vi "SP_BreakDown_Manage.vi"() -> ()   [LabVIEW 2017]
uses:
  <vilib>/addons/database/Connection.llb/DB Tools Open Connec (Path).vi
  Globle/Login Data.vi
  <vilib>/addons/database/NI_Database_API.lvlib
panel:
  in  "Cancel Button - Archive":bool
  out "Stakeholder":string
  out "Role Id":string
  in  "Download 2":bool
  in  "Get Rport 2":bool
  in  "Manage 2":bool
  out "Table 2":string[][](array[string])
  out "error out":errorcluster
  in  "error in (no error)":errorcluster
  out "Table":string[][](table)
  in  "Shift":string(combo)
  in  "Station":string(combo)
  in  "To Date":timestamp format="%<%Y-%m-%d>T"
  in  "From Date":timestamp format="%<%Y-%m-%d>T"
  in  "Stakeholder":string(combo)
  # "Breakdown Manage"
  # "Designed And Developed By - Infinity Automation Systems Pvt. Ltd."
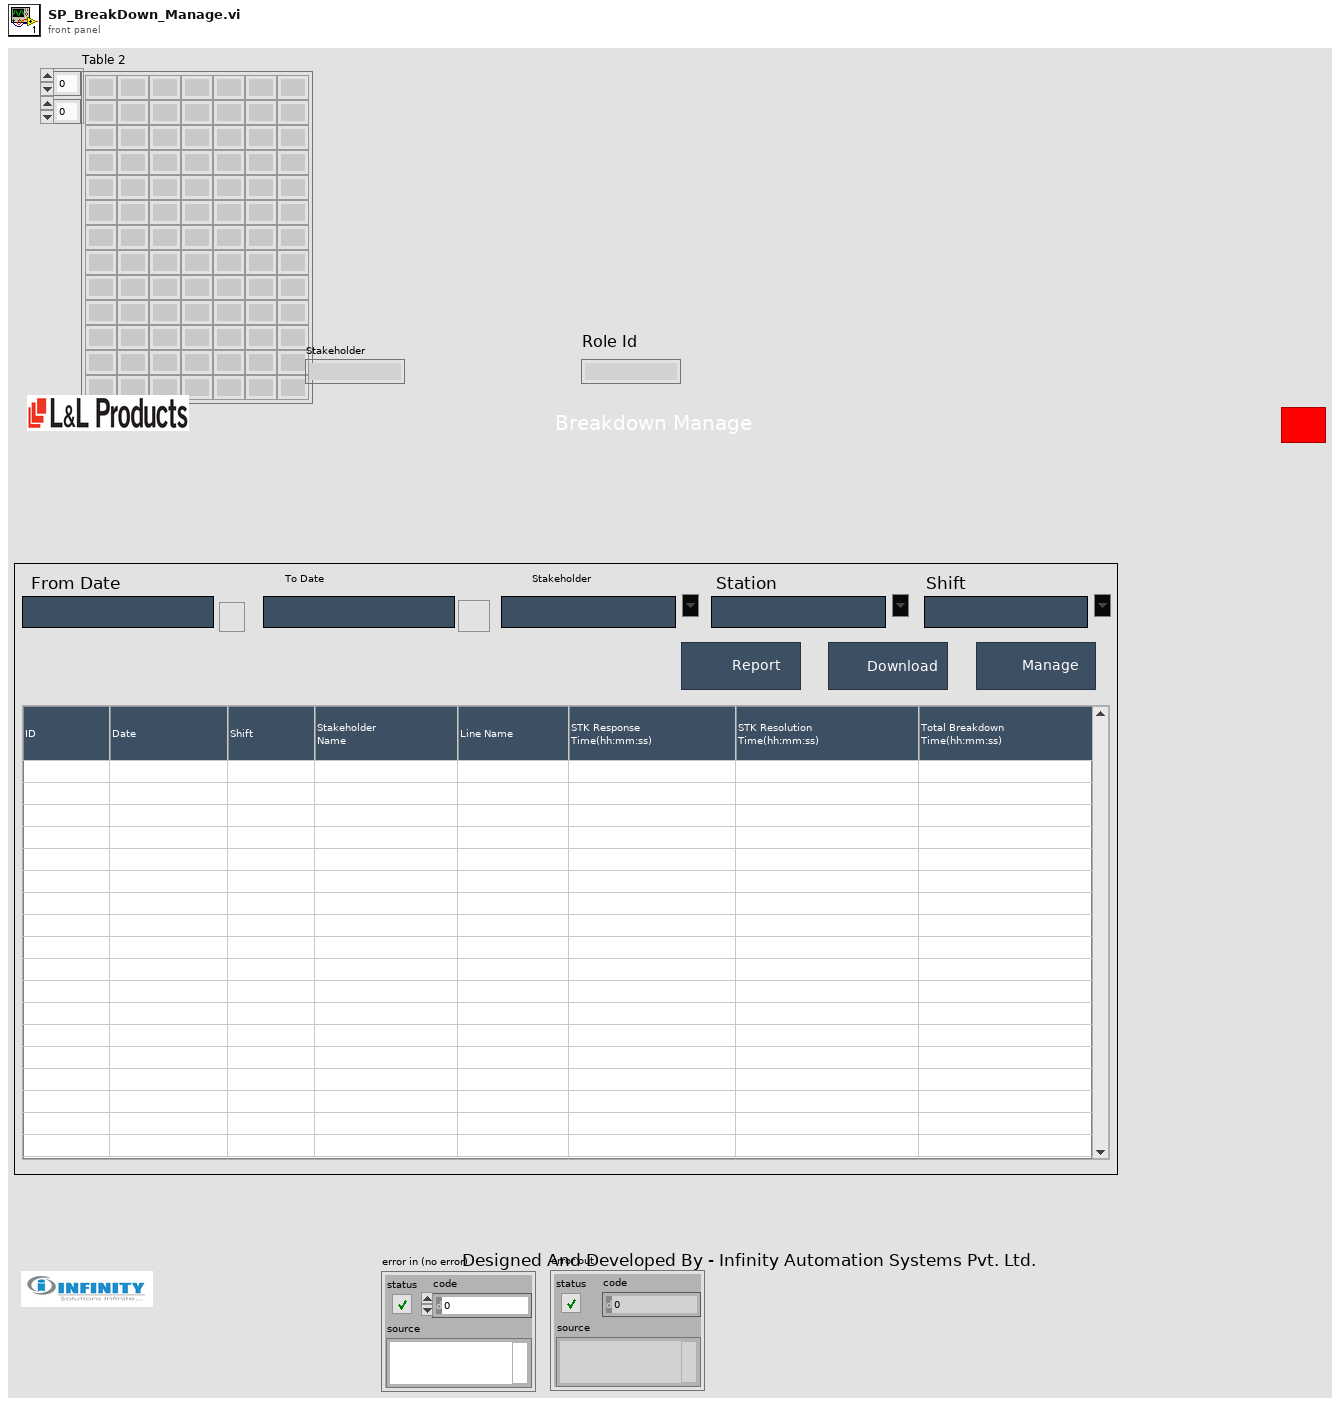
[diagram p1: front panel]
types:
  T1 = typedef "NI_Database_API.lvlib/Conn ObjectReference.ctl" = refnum<k1>
  T2 = enum32{"invalid app kind", "Development System", "Run Time System", "Student Edition", "Embedded LabVIEW", "Evaluation", "Custom"}
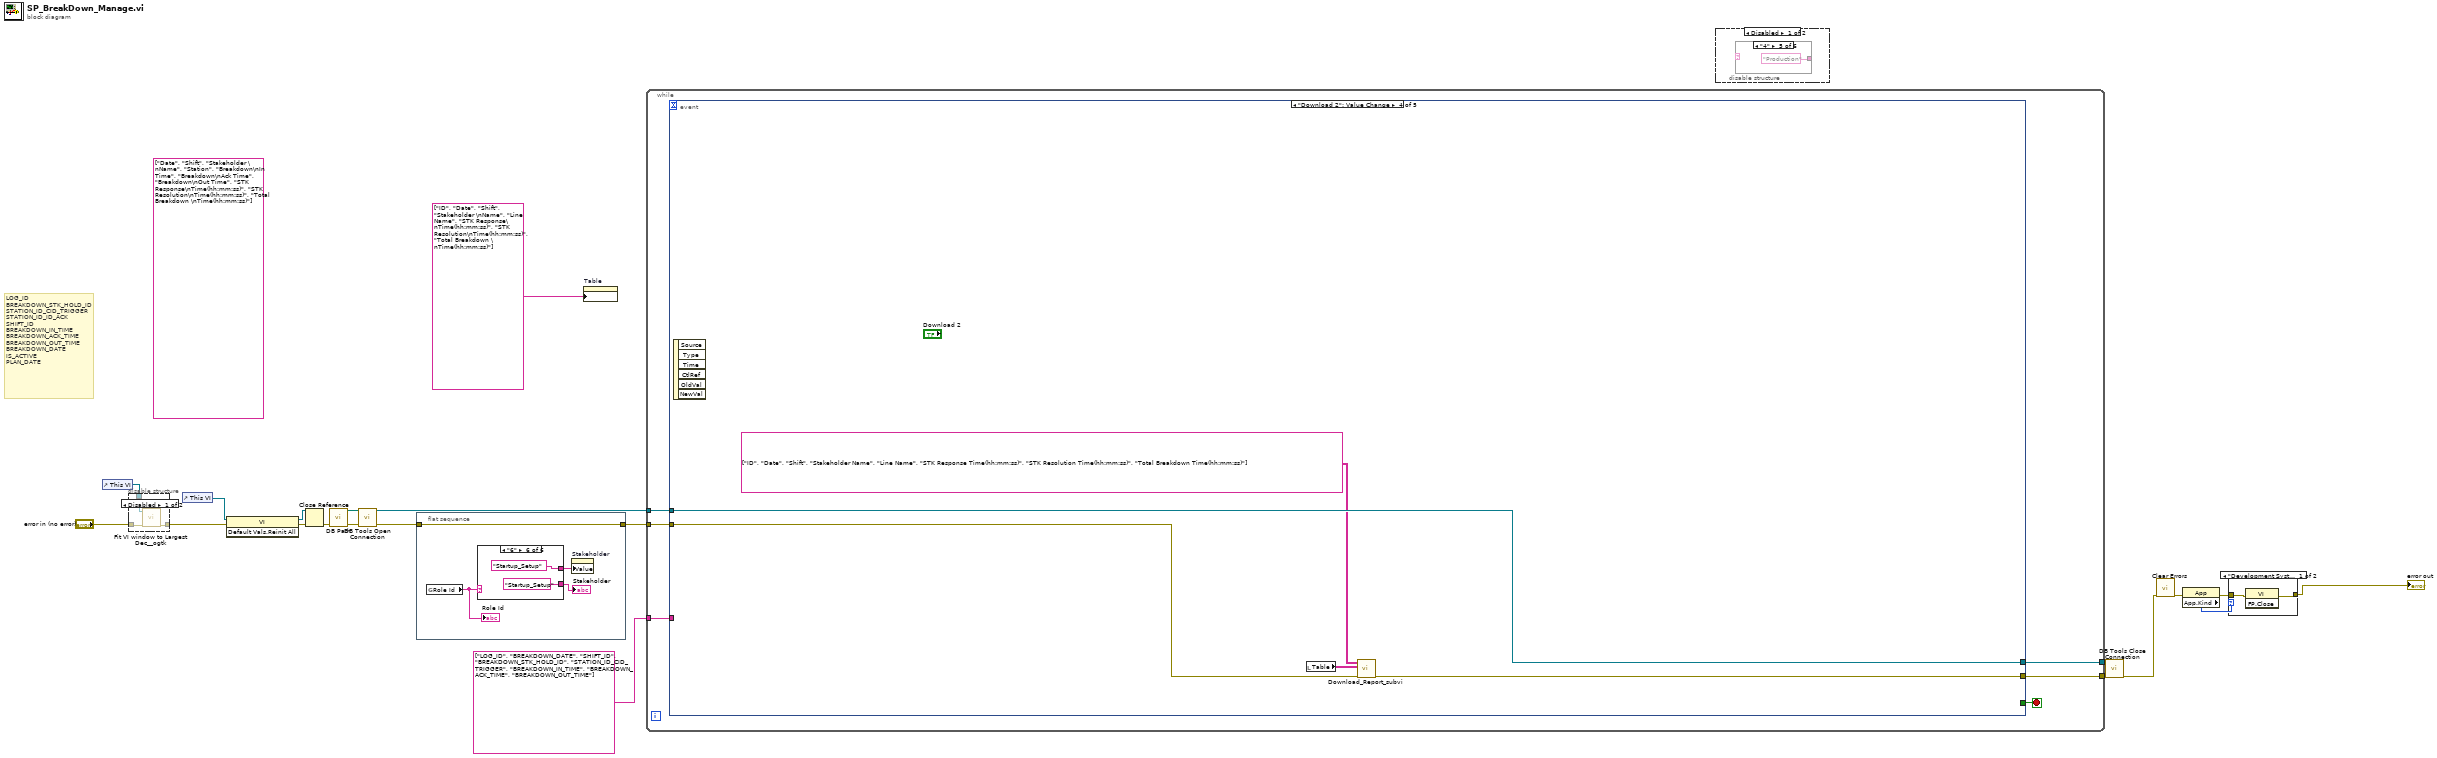
[diagram p0: block diagram]
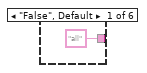
[diagram p2: hidden frame]
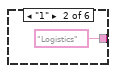
[diagram p3: hidden frame]
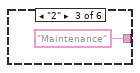
[diagram p4: hidden frame]
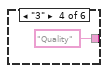
[diagram p5: hidden frame]
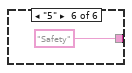
[diagram p6: hidden frame]
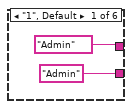
[diagram p8: hidden frame]
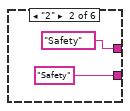
[diagram p9: hidden frame]
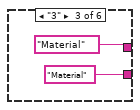
[diagram p10: hidden frame]
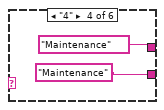
[diagram p11: hidden frame]
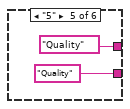
[diagram p12: hidden frame]
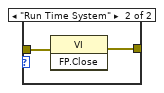
[diagram p13: hidden frame]
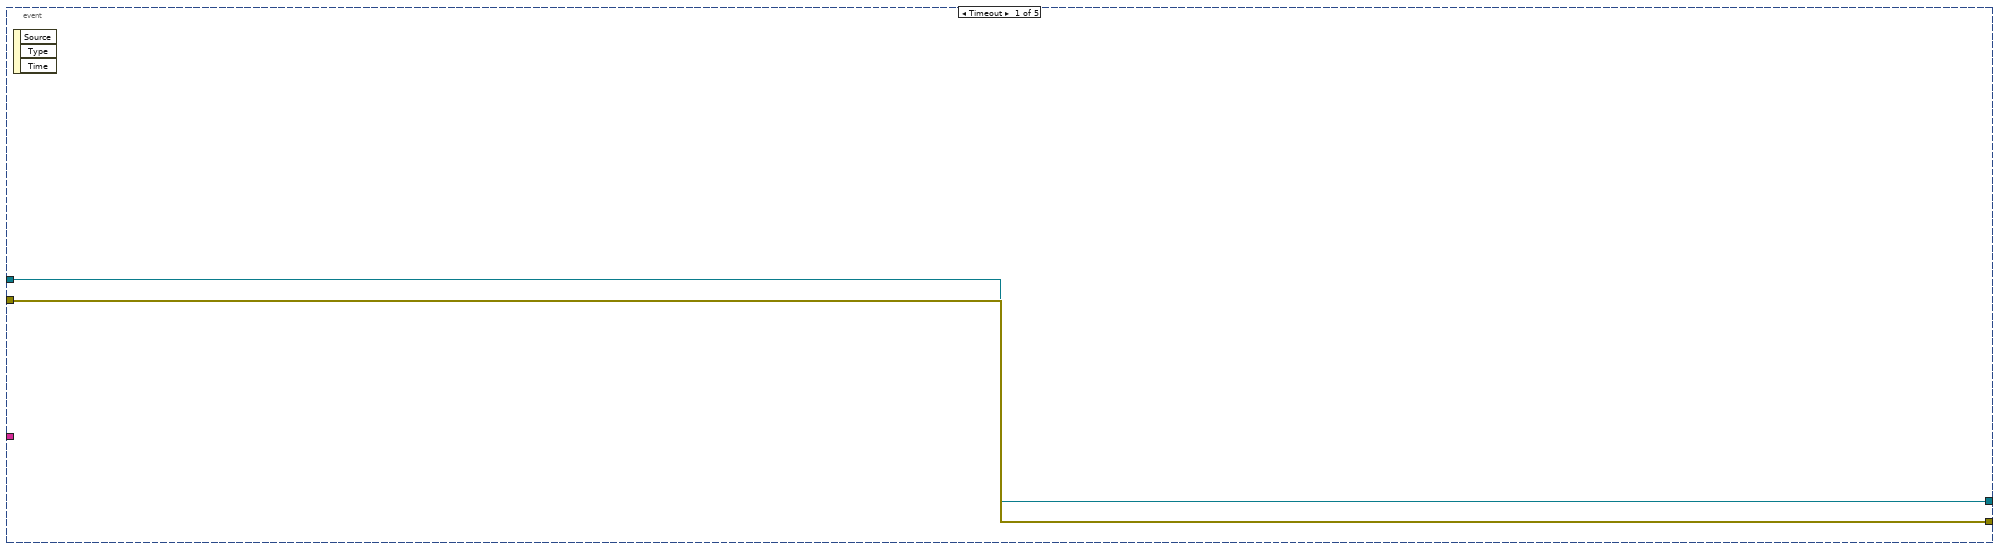
[diagram p14: hidden frame]
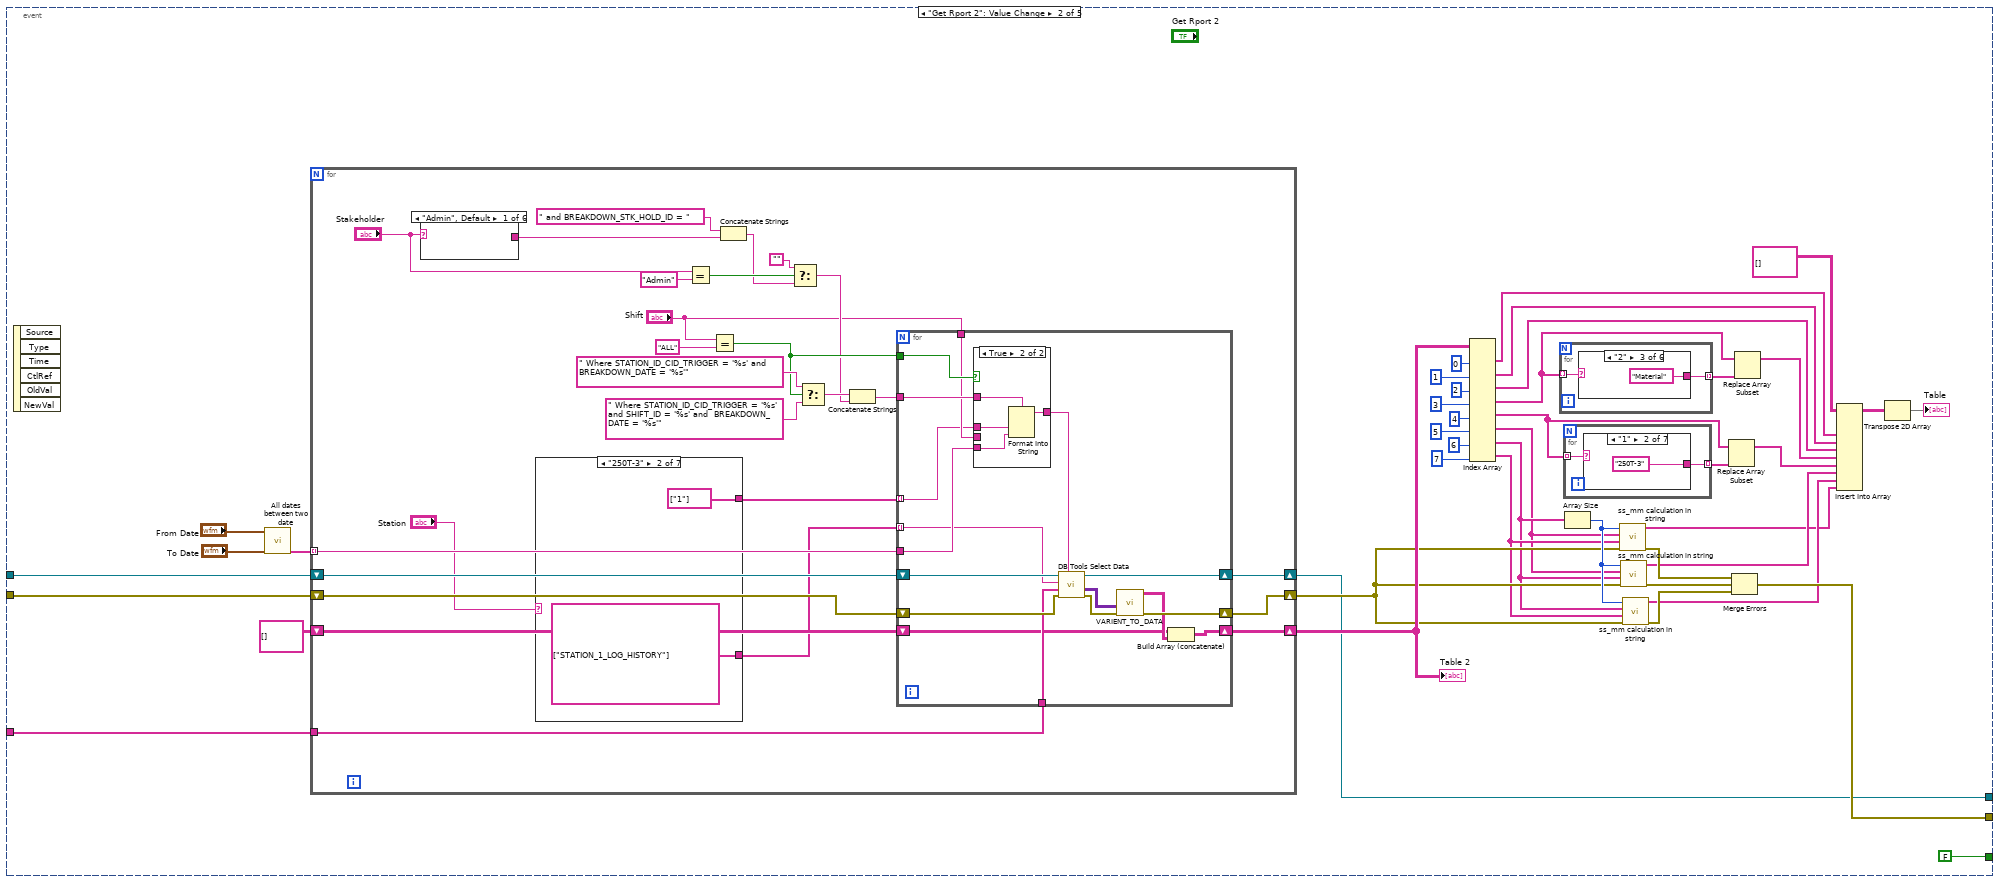
[diagram p15: hidden frame]
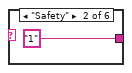
[diagram p16: hidden frame]
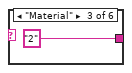
[diagram p17: hidden frame]
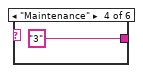
[diagram p18: hidden frame]
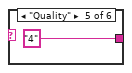
[diagram p19: hidden frame]
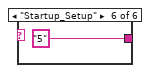
[diagram p20: hidden frame]
diagram:
  (unwired) string[] ["Date", "Shift", "Stakeholder \nName", "Station", "Breakdown\nIn Time", "Breakdown\nAck Time", "Breakdown\nOut Time", "STK Response\nTime(hh:mm:ss)", "STK Resolution\nTime(hh:mm:ss)", "Total Breakdown \nTime(hh:mm:ss)"] ("Column Header Strings[]")
  # "LOG_ID\nBREAKDOWN_STK_HOLD_ID\nSTATION_ID_CID_TRIGGER\nSTATION_ID_ID_ACK\nSHIFT_ID\nBREAKDOWN_IN_TIME\nBREAKDOWN_ACK_TIME\nBREAKDOWN_OUT_TIME\nBREAKDOWN_DATE\nIS_ACTIVE\nPLAN_DATE"
  n1 = control-ref of="This VI"() -> (w10:refnum<vi>)
  n2 = disable-structure shown="Disabled" {
    disable-tunnel: "error in (no error)" -> [w24 _]
    disable-tunnel: [w23 _] -> w11
    disable-tunnel: w10 -> [w22 _]
    frame Disabled {
      n3 = call <userlib>:"Fit VI window to Largest Dec__ogtk.vi"("error in (no error)"=w24, "VI Ref (calling VI)"=w22) -> ("error out"=w23:errorcluster)  [unwired: 4 in, 1 out]
    }
    frame Enabled {
    }
  }
  n4 = control-ref of="This VI"() -> (w21:refnum<vi>)
  n5 = invoke class="VI" method="Default Vals.Reinit All"(reference=w21, error in=w11) -> (reference out=w19:refnum<vi>, error out=w20:errorcluster)  [unwired: 1 in, 1 out]
  n6 = Close Reference(reference=w19, error in (no error)=w20) -> (error out=w18:errorcluster)
  n7 = call "DB Path.vi"("error in"=w18) -> ("error out"=w17:errorcluster, "DB Path"=w16:path)  [unwired: 9 in]
  n8 = call-poly <vilib>:"DB Tools Open Connection.vi"("error in (no error)"=w17, "connection information"=w16) -> ("error out"=w4:errorcluster, "connection reference"=w15:T1)  [unwired: 6 in]
  n9 = flat-sequence {
    tunnel: [w28] -> w3
    tunnel: w4 -> [w28]
    frame #0 {
      n10 = global read "Login Data.vi" "Role Id"() -> (w25:string)
      "Role Id" <- w25
      n11 = case shown="\"6\"" w25 {
        tunnel: ["Admin" ("string") "Safety" "Material" "Maintenance" "Quality" "Startup_Setup"] -> w26
        tunnel: ["Admin" ("Stakeholder") "Safety" ("Stakeholder") "Material" ("Stakeholder") "Maintenance" ("Stakeholder") "Quality" ("Stakeholder") "Startup_Setup" ("Stakeholder")] -> w27
        frame "1", Default {
        }
        frame "2" {
        }
        frame "3" {
        }
        frame "4" {
        }
        frame "5" {
        }
        frame "6" {
        }
      }
      "Stakeholder" <- w26
      n12 = property on="Stakeholder" class="CmbBox"("Value"=w27) -> ()  [unwired: 2 in, 2 out]
    }
  }
  n13 = property on="Table" class="Tbl (strict)"("Column Headers[]"=string[] ["ID", "Date", "Shift", "Stakeholder \nName", "Line Name", "STK Response\nTime(hh:mm:ss)", "STK Resolution\nTime(hh:mm:ss)", "Total Breakdown \nTime(hh:mm:ss)"] ("Column Header Strings[]")) -> ()  [unwired: 2 in, 2 out]
  n14 = while {
    tunnel: w15 -> [w46]
    tunnel: w3 -> [w45]
    tunnel: [w44] -> w14
    tunnel: [w43] -> w13
    tunnel: string[] ["LOG_ID", "BREAKDOWN_DATE", "SHIFT_ID", "BREAKDOWN_STK_HOLD_ID", "STATION_ID_CID_TRIGGER", "BREAKDOWN_IN_TIME", "BREAKDOWN_ACK_TIME", "BREAKDOWN_OUT_TIME"] -> [w42]
    stop <- w41 stop-if-true
    n15 = event shown="[3] \"Download 2\": Value Change" {
      selector: _ -> [_ _ _ _ _]
      dyn-events: _ -> [_ _ _ _ _]
      timeout: _ -> [_ _ _ _ _]
      tunnel: w46 -> [w47 w69 w179 w183 w188]
      tunnel: w45 -> [w48 w68 w181 w186 w189]
      tunnel: [w48 w74 w180 w184 w189] -> w44
      tunnel: [w47 w70 w179 w183 w188] -> w43
      tunnel: w42 -> [_ w67 _ _ _]
      tunnel: [_ FALSE ("Cancel Button - Archive") _ _ "Cancel Button - Archive"] -> w41
      event Timeout {
        n16 = event-data() -> ()  [unwired: 1 in, 3 out]
      }
      event "Get Rport 2": Value Change {
        n17 = event-data() -> ()  [unwired: 1 in, 6 out]
        n18 = call "All dates between two date.vi"("To Date"="To Date", "From Date"="From Date") -> ("All Days (String)"=w66:string[])  [unwired: 8 in, 1 out]
        n19 = for {
          tunnel: w67 -> [w114]
          shift-right: [w109] -> w70
          shift-left: w69 -> [w116]
          shift-right: [w108] -> w71
          shift-left: w68 -> [w115]
          shift-right: [w106] -> w72
          shift-left: string[][] [] -> [w107]
          tunnel: w66 -> [w105] mode=indexing
          n20 = case shown="\"Admin\", Default" "Stakeholder" {
            tunnel: [_ "1" "2" "3" "4" "5"] -> w99
            frame "Admin", Default {
            }
            frame "Safety" {
            }
            frame "Material" {
            }
            frame "Maintenance" {
            }
            frame "Quality" {
            }
            frame "Startup_Setup" {
            }
          }
          n21 = case shown="\"250T-3\"" "Station" {
            tunnel: [string[] ["STATION_1_LOG_HISTORY", "STATION_2_LOG_HISTORY", "STATION_3_LOG_HISTORY", "STATION_4_LOG_HISTORY", "STATION_5_LOG_HISTORY", "STATION_6_LOG_HISTORY"] string[] ["STATION_1_LOG_HISTORY"] string[] ["STATION_2_LOG_HISTORY"] string[] ["STATION_3_LOG_HISTORY"] string[] ["STATION_4_LOG_HISTORY"] string[] ["STATION_5_LOG_HISTORY"] string[] ["STATION_6_LOG_HISTORY"]] -> w104
            tunnel: [string[] ["1", "2", "3", "4", "5", "6"] string[] ["1"] string[] ["2"] string[] ["3"] string[] ["4"] string[] ["5"] string[] ["6"]] -> w103
            frame "ALL", Default {
            }
            frame "250T-3" {
            }
            frame "250T-2" {
            }
            frame "250T-1" {
            }
            frame "400T-1" {
            }
            frame "150T-1" {
            }
            frame "400T-2" {
            }
          }
          n22 = Equal?(x="Stakeholder", y="Admin") -> (x = y?=w101:bool)
          n23 = Equal?(x="Shift", y="ALL" ("x")) -> (x = y?=w110:bool)
          n24 = Concatenate Strings(" and BREAKDOWN_STK_HOLD_ID = " ("format string"), w99) -> (w98:string)
          n25 = Select(t="", s=w101, f=w98) -> (s? t:f=w95:string)
          n26 = Select(t=" Where STATION_ID_CID_TRIGGER = '%s' and BREAKDOWN_DATE = '%s'" ("format string"), s=w110, f=" Where STATION_ID_CID_TRIGGER = '%s' and SHIFT_ID = '%s' and  BREAKDOWN_DATE = '%s'" ("format string")) -> (s? t:f=w96:string)
          n27 = Concatenate Strings(w96, w95) -> (w94:string)
          n28 = for {
            tunnel: w114 -> [w150]
            tunnel: w105 -> [w144]
            tunnel: w94 -> [w147]
            tunnel: w110 -> [w146]
            tunnel: w104 -> [w137] mode=indexing
            tunnel: "Shift" -> [w145]
            shift-right: [w142] -> w108
            shift-left: w115 -> [w151]
            shift-right: [w141] -> w109
            shift-left: w116 -> [w152]
            shift-right: [w138] -> w106
            shift-left: w107 -> [w139]
            tunnel: w103 -> [w136] mode=indexing
            n29 = case shown="True" w146 {
              tunnel: w147 -> [w157 w161]
              tunnel: w136 -> [w156 w160]
              tunnel: w145 -> [w154 _]
              tunnel: w144 -> [w153 w158]
              tunnel: [w155 w159] -> w143
              frame False {
                n30 = Format Into String(format string=w157, w156, w154, w153) -> (resulting string=w155:string)  [unwired: 2 in, 1 out]
              }
              frame True {
                n31 = Format Into String(format string=w161, w160, w158) -> (resulting string=w159:string)  [unwired: 2 in, 1 out]
              }
            }
            n32 = call <vilib>:"DB Tools Select Data.vi"("condition"=w143, "error in (no error)"=w151, "columns"=w150, "table"=w137, "connection reference"=w152) -> ("error out"=w148:errorcluster, "data"=w149:variant[][], "connection reference out"=w141:T1)  [unwired: 1 in]
            n33 = call "VARIENT_TO_DATA.vi"("data"=w149, "error in (no error)"=w148) -> ("Table"=w140:string[][], "error out"=w142:errorcluster)  [unwired: 7 in]
            n34 = Build Array (concatenate)(w139, w140) -> (w138:string[][])
          }
        }
        "Table 2" <- w72
        n35 = Index Array(array=w72, index (col) #1=0 ("disabled index (col)"), index (col) #2=1 ("disabled index (col)"), index (col) #3=2 ("disabled index (col)"), index (col) #4=3 ("disabled index (col)"), index (col) #5=4 ("disabled index (col)"), index (col) #6=5 ("disabled index (col)"), index (col) #7=6 ("disabled index (col)"), index (col) #8=7 ("disabled index (col)")) -> (element #1=w54:string[], element #2=w53:string[], element #3=w52:string[], element #4=w55:string[], element #5=w56:string[], element #6=w57:string[], element #7=w58:string[], element #8=w59:string[])  [unwired: 8 in]
        n36 = for {
          tunnel: w55 -> [w172] mode=indexing
          tunnel: [w171] -> w88 mode=indexing
          n37 = case shown="\"2\"" w172 {
            tunnel: ["all" "Safety" "Material" "Maintenance" "Quality" "Startup_Setup"] -> w171
            frame "False", Default {
            }
            frame "1" {
            }
            frame "2" {
            }
            frame "3" {
            }
            frame "4" {
            }
            frame "5" {
            }
          }
        }
        n38 = for {
          tunnel: w56 -> [w163] mode=indexing
          tunnel: [w162] -> w86 mode=indexing
          n39 = case shown="\"1\"" w163 {
            tunnel: ["ALL" "250T-3" "250T-2" "250T-1" "400T-1" "150T-1" "400T-2"] -> w162
            frame "ALL", Default {
            }
            frame "1" {
            }
            frame "2" {
            }
            frame "3" {
            }
            frame "4" {
            }
            frame "5" {
            }
            frame "6" {
            }
          }
        }
        n40 = Array Size(array=w58) -> (size(s)=w78:i32)
        n41 = call "ss_mm calculation in string.vi"("error in (no error)"=w71, "Table 2"=w59, "Table"=w57, "Numeric"=w78) -> ("error out"=w77:errorcluster, "Array 2"=w49:string[])  [unwired: 6 in]
        n42 = call "ss_mm calculation in string.vi"("error in (no error)"=w71, "Table 2"=w58, "Table"=w57, "Numeric"=w78) -> ("error out"=w76:errorcluster, "Array 2"=w51:string[])  [unwired: 6 in]
        n43 = call "ss_mm calculation in string.vi"("error in (no error)"=w71, "Table 2"=w59, "Table"=w58, "Numeric"=w78) -> ("error out"=w75:errorcluster, "Array 2"=w50:string[])  [unwired: 6 in]
        n44 = Replace Array Subset(array=w56, new element=w86) -> (w61:string[])  [unwired: 1 in]
        n45 = Merge Errors(w77, w76, w75) -> (w74:errorcluster)
        n46 = Replace Array Subset(array=w55, new element=w88) -> (w62:string[])  [unwired: 1 in]
        n47 = Insert Into Array(array=string[][] [], new element #1=w54, new element #2=w53, new element #3=w52, new element #4=w62, new element #5=w61, new element #6=w51, new element #7=w50, new element #8=w49) -> (w80:string[][])  [unwired: 2 in]
        n48 = Transpose 2D Array(2D array=w80) -> (transposed array=→"Table":string[][])
      }
      event "Manage 2": Value Change {
        n49 = event-data() -> ()  [unwired: 1 in, 6 out]
        n50 = call "manage breakdown sub.vi"("error in (no error)"=w181) -> ("error out"=w180:errorcluster)  [unwired: 10 in]
      }
      event "Download 2": Value Change {
        n51 = event-data() -> ()  [unwired: 1 in, 6 out]
        n52 = local read "Table"() -> (w185:string[][])
        n53 = call "Download_Report_subvi.vi"("error in (no error)"=w186, "Value"=w185, "Column Header Strings[]"=string[][] [["ID", "Date", "Shift", "Stakeholder Name", "Line Name", "STK Response Time(hh:mm:ss)", "STK Resolution Time(hh:mm:ss)", "Total Breakdown Time(hh:mm:ss)"]]) -> ("error out"=w184:errorcluster)  [unwired: 8 in]
      }
      event "Cancel Button - Archive": Value Change {
        n54 = event-data() -> ()  [unwired: 1 in, 6 out]
      }
    }
  }
  n55 = disable-structure shown="Disabled" {
    frame Disabled {
      n56 = case shown="\"4\"" {
        selector: _ -> [_ _ _ _ _ _]
        tunnel: ["all" "Logistics" "Maintenance" "Quality" "Production" "Safety"] -> _
        frame "False", Default {
        }
        frame "1" {
        }
        frame "2" {
        }
        frame "3" {
        }
        frame "4" {
        }
        frame "5" {
        }
      }
    }
    frame Enabled {
    }
  }
  n57 = call <vilib>:"DB Tools Close Connection.vi"("error in (no error)"=w14, "connection reference"=w13) -> ("error out"=w6:errorcluster)  [unwired: 5 in]
  n58 = call <vilib>:"Clear Errors.vi"("error in (no error)"=w6) -> ("error out"=w9:errorcluster)  [unwired: 5 in, 1 out]
  n59 = property class="App"(error in=w9) -> (error out=w8:errorcluster, "App.Kind"=w7:T2)  [unwired: 1 in, 1 out]
  n60 = case shown="\"Development System\", Default" w7 {
    tunnel: w8 -> [w197 w199]
    tunnel: [w196 w198] -> w5
    frame "Development System", Default {
      n61 = invoke class="VI" method="FP.Close"(error in=w197) -> (error out=w196:errorcluster)  [unwired: 2 in, 2 out]
    }
    frame "Run Time System" {
      n62 = invoke class="VI" method="FP.Close"(error in=w199) -> (error out=w198:errorcluster)  [unwired: 2 in, 2 out]
    }
  }
  "error out" <- w5
